vi "Get Thermal Information.vi"(8 "error in":errorcluster, 10 "LDO Input":string[][](array[string]), 11 "PLC Data In":T1) -> (0 "error out":errorcluster, 2 "LDO Output":string[][](array[string]), 3 "PLC Data Out":T1)   [LabVIEW 2020]
uses:
  Modbus/Modbus PLC Data All.ctl
  Modbus/Modbus FVIR Control.ctl
  Modbus/Modbus LDO Control.ctl
  WritingDataFile/Data to Save.ctl
panel:
  in  "Constant Thermal Eff":dbl format="%#.5g"
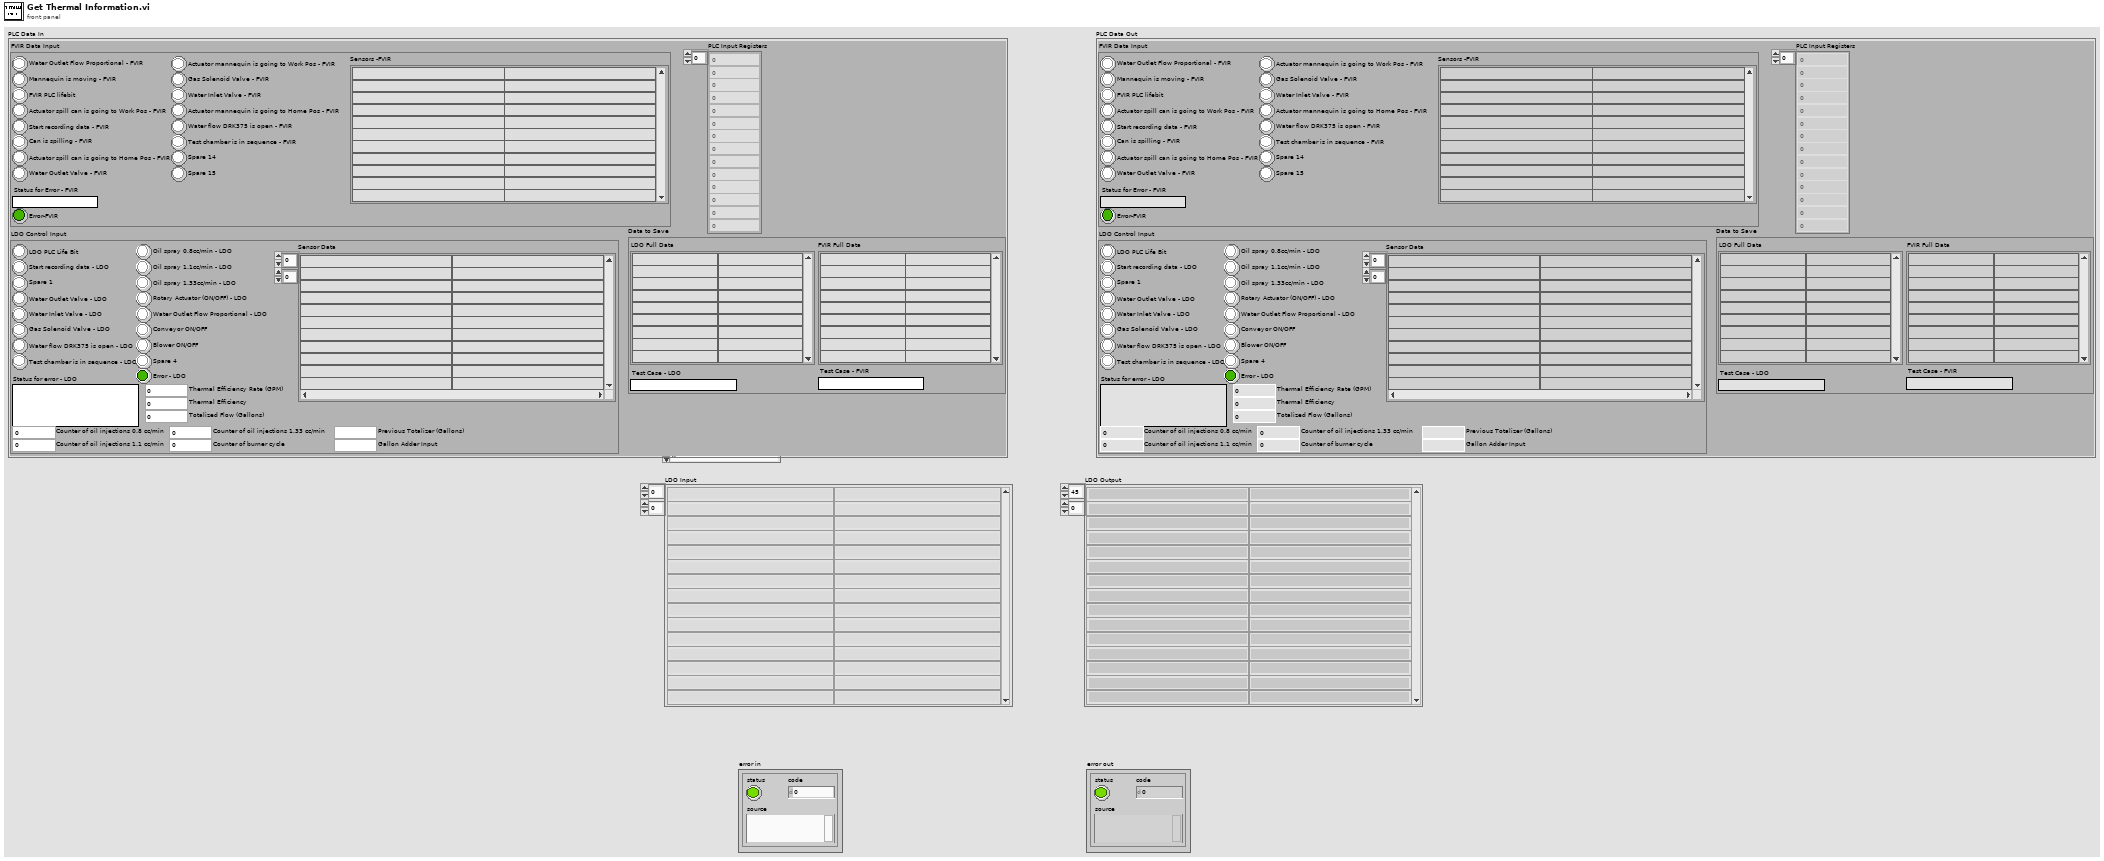
[diagram p1: front panel]
types:
  T1 = typedef "Modbus PLC Data All.ctl" = cluster{"FVIR Data Input":T2, "LDO Control Input":T3, "PLC Input Registers":i16[], "Data to Save":T4}
  T2 = typedef "Modbus FVIR Control.ctl" = cluster{"Spare 15":bool, "Spare 14":bool, "Actuator mannequin is going to Work Pos - FVIR":bool, "Actuator mannequin is going to Home Pos - FVIR":bool, "Test chamber is in sequence - FVIR ":bool, "Water flow DRK375 is open - FVIR":bool, "Gas Solenoid Valve - FVIR":bool, "Water Inlet Valve - FVIR":bool, "Water Outlet Flow Proportional - FVIR":bool, "Start recording data - FVIR":bool, "Actuator spill can is going to Work Pos - FVIR":bool, "Actuator spill can is going to Home Pos - FVIR":bool, "Water Outlet Valve - FVIR":bool, "Can is spilling - FVIR":bool, "Mannequin is moving - FVIR":bool, "FVIR PLC lifebit":bool, "Status for Error - FVIR":string, "Error-FVIR":bool, "Sensors -FVIR":string[][]}
  T3 = typedef "Modbus LDO Control.ctl" = cluster{"LDO PLC Life Bit":bool, "Start recording data - LDO":bool, "Spare 1":bool, "Water Outlet Valve - LDO":bool, "Water Inlet Valve - LDO":bool, "Gas Solenoid Valve - LDO":bool, "Water flow DRK375 is open - LDO":bool, "Test chamber is in sequence - LDO":bool, "Oil spray 0.8cc/min - LDO":bool, "Oil spray 1.1cc/min - LDO":bool, "Oil spray 1.33cc/min - LDO":bool, "Rotary Actuator (ON/OFF) - LDO":bool, "Water Outlet Flow Proportional - LDO":bool, "Conveyor ON/OFF":bool, "Blower ON/OFF":bool, "Spare 4":bool, "Status for error - LDO":string, "Error - LDO":bool, "Sensor Data":string[][], "Thermal Efficiency Rate (GPM)":dbl, "Thermal Efficiency":dbl, "Totalized Flow (Gallons)":dbl, "Counter of oil injections 1.33 cc/min":u16, "Counter of burner cycle":u16, "Counter of oil injections 1.1 cc/min":u16, "Counter of oil injections 0.8 cc/min":u16, "Previous Totalizer (Gallons)":dbl, "Gallon Adder Input":dbl}
  T4 = typedef "Data to Save.ctl" = cluster{"LDO Full Data":string[][], "FVIR Full Data":string[][], "Test Case - FVIR":string, "Test Case - LDO":string}
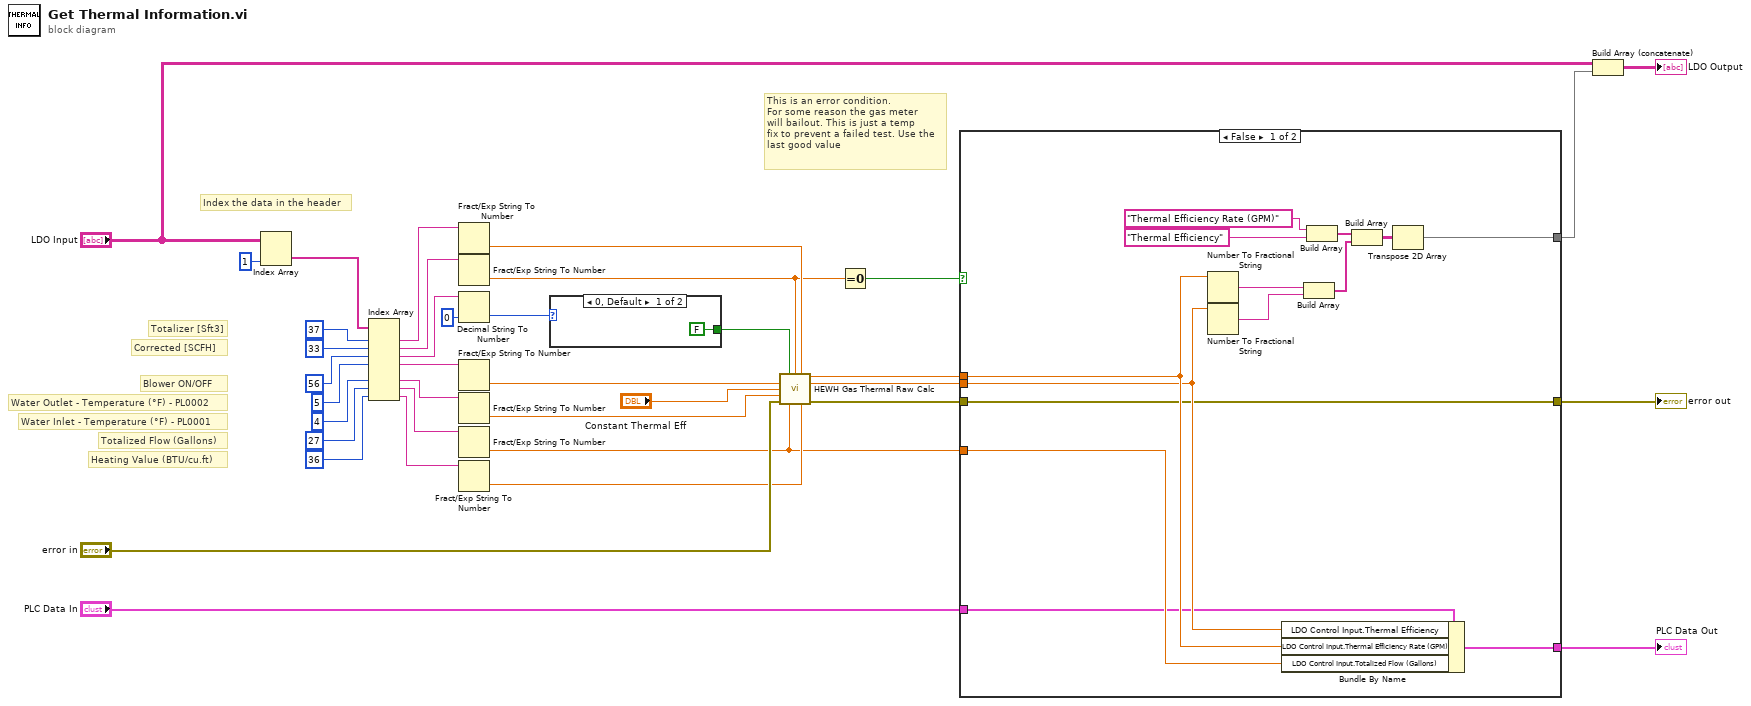
[diagram p0: block diagram]
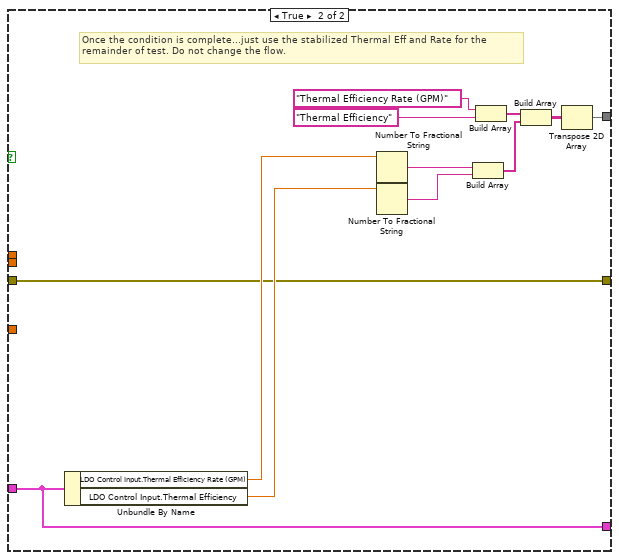
[diagram p2: hidden frame]
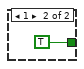
[diagram p3: hidden frame]
diagram:
  # "This is an error condition.\nFor some reason the gas meter \nwill bailout. This is just a temp\nfix to prevent a failed test. Use the\nlast good value"
  # "Blower ON/OFF"
  # "Totalizer [Sft3]"
  # "Corrected [SCFH]"
  # "Heating Value (BTU/cu.ft)"
  # "Totalized Flow (Gallons)"
  # "Water Outlet - Temperature (°F) - PL0002"
  # "Water Inlet - Temperature (°F) - PL0001"
  # "Index the data in the header"
  n1 = Index Array(array="LDO Input", index (col)=1 ("disabled index (col)")) -> (element=w34:string[])  [unwired: 1 in]
  n2 = Index Array(array=w34, index #1=37 ("index"), index #2=33 ("index"), index #3=56 ("index"), index #4=5 ("index"), index #6=4 ("index"), index #7=27 ("index"), index #8=36 ("index")) -> (element #1=w29:string, element #2=w30:string, element #3=w16:string, element #4=w19:string, element #6=w20:string, element #7=w21:string, element #8=w22:string)  [unwired: 1 in, 1 out]
  n3 = Fract/Exp String To Number(string=w29) -> (number=w26:dbl)  [unwired: 3 in, 1 out]
  n4 = Fract/Exp String To Number(string=w30) -> (number=w2:dbl)  [unwired: 3 in, 1 out]
  n5 = Decimal String To Number(string=w16, default (0L)=u8 0) -> (number=w14:u8)  [unwired: 1 in, 1 out]
  n6 = Fract/Exp String To Number(string=w19) -> (number=w33:dbl)  [unwired: 3 in, 1 out]
  n7 = Fract/Exp String To Number(string=w20) -> (number=w32:dbl)  [unwired: 3 in, 1 out]
  n8 = Fract/Exp String To Number(string=w21) -> (number=w6:dbl)  [unwired: 3 in, 1 out]
  n9 = Fract/Exp String To Number(string=w22) -> (number=w31:dbl)  [unwired: 3 in, 1 out]
  n10 = case shown="0, Default" w14 {
    tunnel: [FALSE TRUE] -> w13
    frame 0, Default {
    }
    frame 1 {
    }
  }
  n11 = call "HEWH Gas Thermal Raw Calc.vi"("Use Constant Thermal Efficiency"=w13, "Gas Mass Flow"=w2, "Gas Totalizer"=w26, "RTD Out (Deg F)"=w33, "Constant Thermal Eff"="Constant Thermal Eff", "RTD In (Deg F)"=w32, "error in (no error)"="error in", "Gallons (Gal)"=w6, "Gross Heating Value, Vol (Real, Dry)"=w31) -> ("Rate"=w9:dbl, "Eff"=w7:dbl, "error out"=w4:errorcluster)  [unwired: 4 in]
  n12 = Equal To 0?(x=w2) -> (x = 0?=w1:bool)
  n13 = case shown="False" w1 {
    tunnel: [w46 w55] -> w10
    tunnel: w9 -> [w45 _]
    tunnel: [w44 w65] -> w8
    tunnel: w7 -> [w43 _]
    tunnel: w6 -> [w42 _]
    tunnel: "PLC Data In" -> [w41 w65]
    tunnel: w4 -> [w40 w54]
    tunnel: [w40 w54] -> w3
    frame False {
      n14 = Number To Fractional String(number=w45) -> (F-format string=w53:string)  [unwired: 3 in]
      n15 = Number To Fractional String(number=w43) -> (F-format string=w52:string)  [unwired: 3 in]
      n16 = Bundle By Name(cluster=w41, "LDO Control Input.Thermal Efficiency"=w43, "LDO Control Input.Thermal Efficiency Rate (GPM)"=w45, "LDO Control Input.Totalized Flow (Gallons)"=w42) -> (w44:T1)
      n17 = Build Array(w53, w52) -> (w49:string[])
      n18 = Build Array("Thermal Efficiency Rate (GPM)", "Thermal Efficiency") -> (w48:string[])
      n19 = Build Array(w48, w49) -> (w47:string[][])
      n20 = Transpose 2D Array(2D array=w47) -> (transposed array=w46:string[][])
    }
    frame True {
      # "Once the condition is complete...just use the stabilized Thermal Eff and Rate for the \nremainder of test. Do not change the flow."
      n21 = Unbundle By Name(w65) -> ("LDO Control Input.Thermal Efficiency Rate (GPM)"=w57:dbl, "LDO Control Input.Thermal Efficiency"=w56:dbl)
      n22 = Number To Fractional String(number=w57) -> (F-format string=w64:string)  [unwired: 3 in]
      n23 = Number To Fractional String(number=w56) -> (F-format string=w63:string)  [unwired: 3 in]
      n24 = Build Array(w64, w63) -> (w62:string[])
      n25 = Build Array("Thermal Efficiency Rate (GPM)", "Thermal Efficiency") -> (w61:string[])
      n26 = Build Array(w61, w62) -> (w60:string[][])
      n27 = Transpose 2D Array(2D array=w60) -> (transposed array=w55:string[][])
    }
  }
  "error out" <- w3
  "PLC Data Out" <- w8
  n28 = Build Array (concatenate)("LDO Input", w10) -> (→"LDO Output":string[][])
